vi "getQuantity.vi"(8 "error in (no error)":errorcluster, 11 "IUnit in":refnum<class "IUnit.lvclass">) -> (0 "error out":errorcluster, 2 "Quantity out":string, 3 "IUnit out":refnum<class "IUnit.lvclass">)   [LabVIEW 2022 SP3, in "openDAQ.lvlib" / "IBaseObject.lvlib" / "IUnit.lvlib" / "IUnit.lvclass"]
uses:
  <instrlib>/openDAQ/Public/Classes/IUnit/IUnit.lvclass
  <instrlib>/openDAQ/Public/Classes/IUnit/IUnit.lvclass/IUnit.ctl
  <instrlib>/openDAQ/Public/Classes/daqCoreTypes/IString/IString.lvclass
  <instrlib>/openDAQ/Binaries/Windows/x86/copendaq32.dll
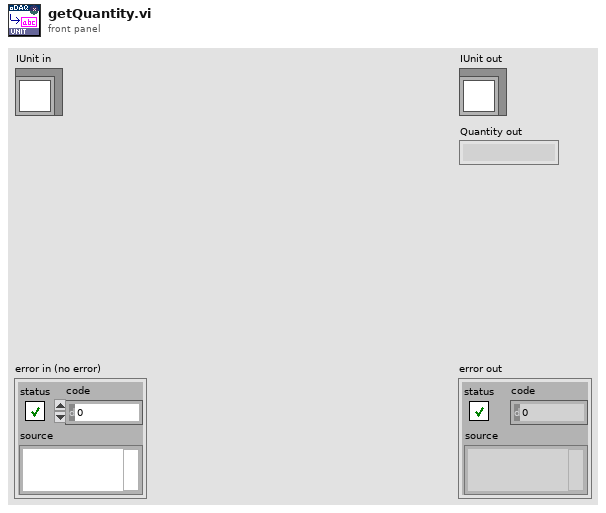
[diagram p1: front panel]
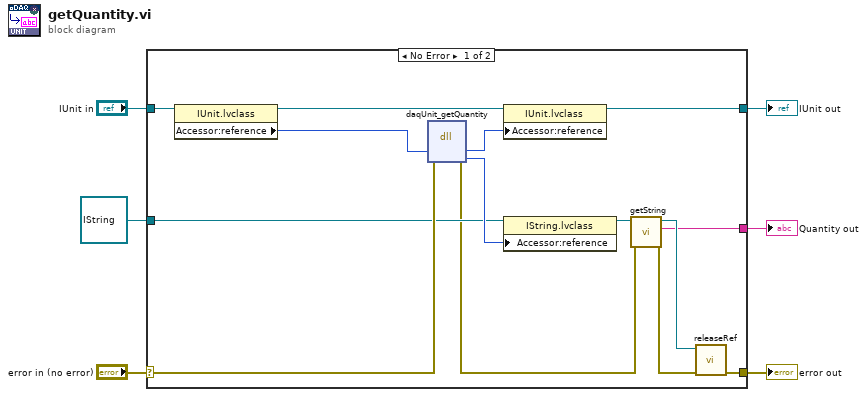
[diagram p0: block diagram]
diagram:
  n1 = case shown="No Error" "error in (no error)" {
    selector: "error in (no error)" -> [w18 w22]
    tunnel: [w8 w22] -> w5
    tunnel: [w15 w21] -> w3
    tunnel: "IUnit in" -> [w19 w21]
    tunnel: refnum<class "IString.lvclass"> refnum ("openDAQ.lvlib:daqCoreTypes.lvlib:IString.lvclass") -> [w13 _]
    tunnel: [w7 _] -> w1
    frame No Error {
      n2 = property class="IUnit.lvclass"(reference=w19) -> (reference out=w16:refnum<class "IUnit.lvclass">, "Accessor:reference"=w17:i64)  [unwired: 1 in, 1 out]
      n3 = dll-call lib="C:/Program Files (x86)/National Instruments/LabVIEW 2022/instr.lib/openDAQ/Binaries/Windows/x86/copendaq*.*" fn="daqUnit_getQuantity"(error in=w18, "unit"=w17) -> (error out=w11:errorcluster, "unit"=w14:i64, "quantity"=w20:i64)  [unwired: 4 in, 1 out]
      n4 = property class="IUnit.lvclass"(reference=w16, "Accessor:reference"=w14) -> (reference out=w15:refnum<class "IUnit.lvclass">)  [unwired: 1 in, 1 out]
      n5 = property class="IString.lvclass"(reference=w13, "Accessor:reference"=w20) -> (reference out=w12:refnum<class "IString.lvclass">)  [unwired: 1 in, 1 out]
      n6 = call <instrlib>:"getString.vi"("error in (no error)"=w11, "IString in"=w12) -> ("error out"=w9:errorcluster, "String out"=w7:string, "IString out"=w10:refnum<class "IString.lvclass">)  [unwired: 7 in]
      n7 = call-dynamic "releaseRef.vi"("error in (no error)"=w9, "IBaseObject in"=w10) -> ("error out"=w8:errorcluster)  [unwired: 9 in]
    }
    frame Error {
    }
  }
  "error out" <- w5
  "IUnit out" <- w3
  "Quantity out" <- w1
